vi "GetLowPrioritySensors.vi"() -> ()   [LabVIEW 2020]
doc: "All low priority sensor reads should be placed in this VI."
uses:
  GlobalMiscellaneous.vi
  GlobalDriverStationData.vi
  GlobalDrivebase.vi
  GRNF_CTREMotor.vi
  <vilib>/Rock Robotics/WPI/ThirdParty/Phoenix-LabVIEW/Motor Controller/Get/CTRE_Phoenix_MotorController_GetTemperature.vi
  GRNF_Compressor.vi
panel:
  out "Pressure Change (psi/min)":dbl
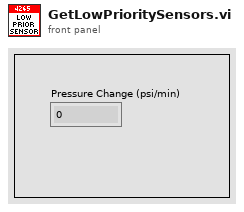
[diagram p1: front panel]
types:
  T1 = typedef "WPI_MotorControlDeviceRef.ctl" = cluster{"DeviceStatus":errorcluster, "Type":T2, "PWM":cluster{"PWM Channel":T3, "DeadBand":T4}, "CAN":cluster{"Device Number":u8, "SetOutput VI Ref":variant, "GetOutput VI Ref":variant, "Enable VI Ref":variant, "Disable VI Ref":variant, "Data":variant}, "Invert":bool, "DIO PWM":cluster{"PWM \"Enable\" Channel":T3, "DIOChannel":T5, "PWM Rate":dbl}}
  T2 = typedef "WPI_MotorControlType.ctl" = enum16{"PWM", "CAN", "DIO PWM"}
  T3 = typedef "FPGA_DIOPWMChannel.ctl" = enum8{"PWM 0", "PWM 1", "PWM 2", "PWM 3", "PWM 4", "PWM 5", "PWM 6", "PWM 7", "PWM 8", "PWM 9", "PWM MXP 0", "PWM MXP 1", "PWM MXP 2", "PWM MXP 3", "PWM MXP 4", "PWM MXP 5", "PWM MXP 6", "PWM MXP 7", "PWM MXP 8", "PWM MXP 9", "Invalid"}
  T4 = typedef "WPI_PWMDeadband.ctl" = cluster{"Name":string, "maxPositivePwm":i32, "minPositivePwm":i32, "centerPwm":i32, "maxNegativePwm":i32, "minNegativePwm":i32, "angularRange":u16}
  T5 = typedef "FPGA_DIOChannel.ctl" = enum8{"DIO 0", "DIO 1", "DIO 2", "DIO 3", "DIO 4", "DIO 5", "DIO 6", "DIO 7", "DIO 8", "DIO 9", "DIO MXP 0", "DIO MXP 1", "DIO MXP 2", "DIO MXP 3", "DIO MXP 4", "DIO MXP 5", "DIO MXP 6", "DIO MXP 7", "DIO MXP 8", "DIO MXP 9", "DIO MXP 10", "DIO MXP 11", "DIO MXP 12", "DIO MXP 13", "DIO MXP 14", "DIO MXP 15", "SPI Port CS1", "SPI Port CS2", "SPI Port CS3", "SPI Port MISO", "SPI Port MOSI", "Invalid"}
  T6 = typedef "WPI_CompressorDevRef.ctl" = cluster{"DevStatus":errorcluster, "Pneumatics Control Module":u8}
  T7 = cluster{"Pressure 0 (psi)":dbl, "Pressure 1 (psi)":dbl}
  T8 = cluster{"Battery Voltage Fault":bool, "Hardware Fault":bool, "CAN Warning Fault":bool, "Temperature Fault":bool}
  T9 = cluster{"HardwareFault":bool, "CompressorFault":bool, "SolenoidFault":bool, "Compressor Open":bool, "Brownout":bool}
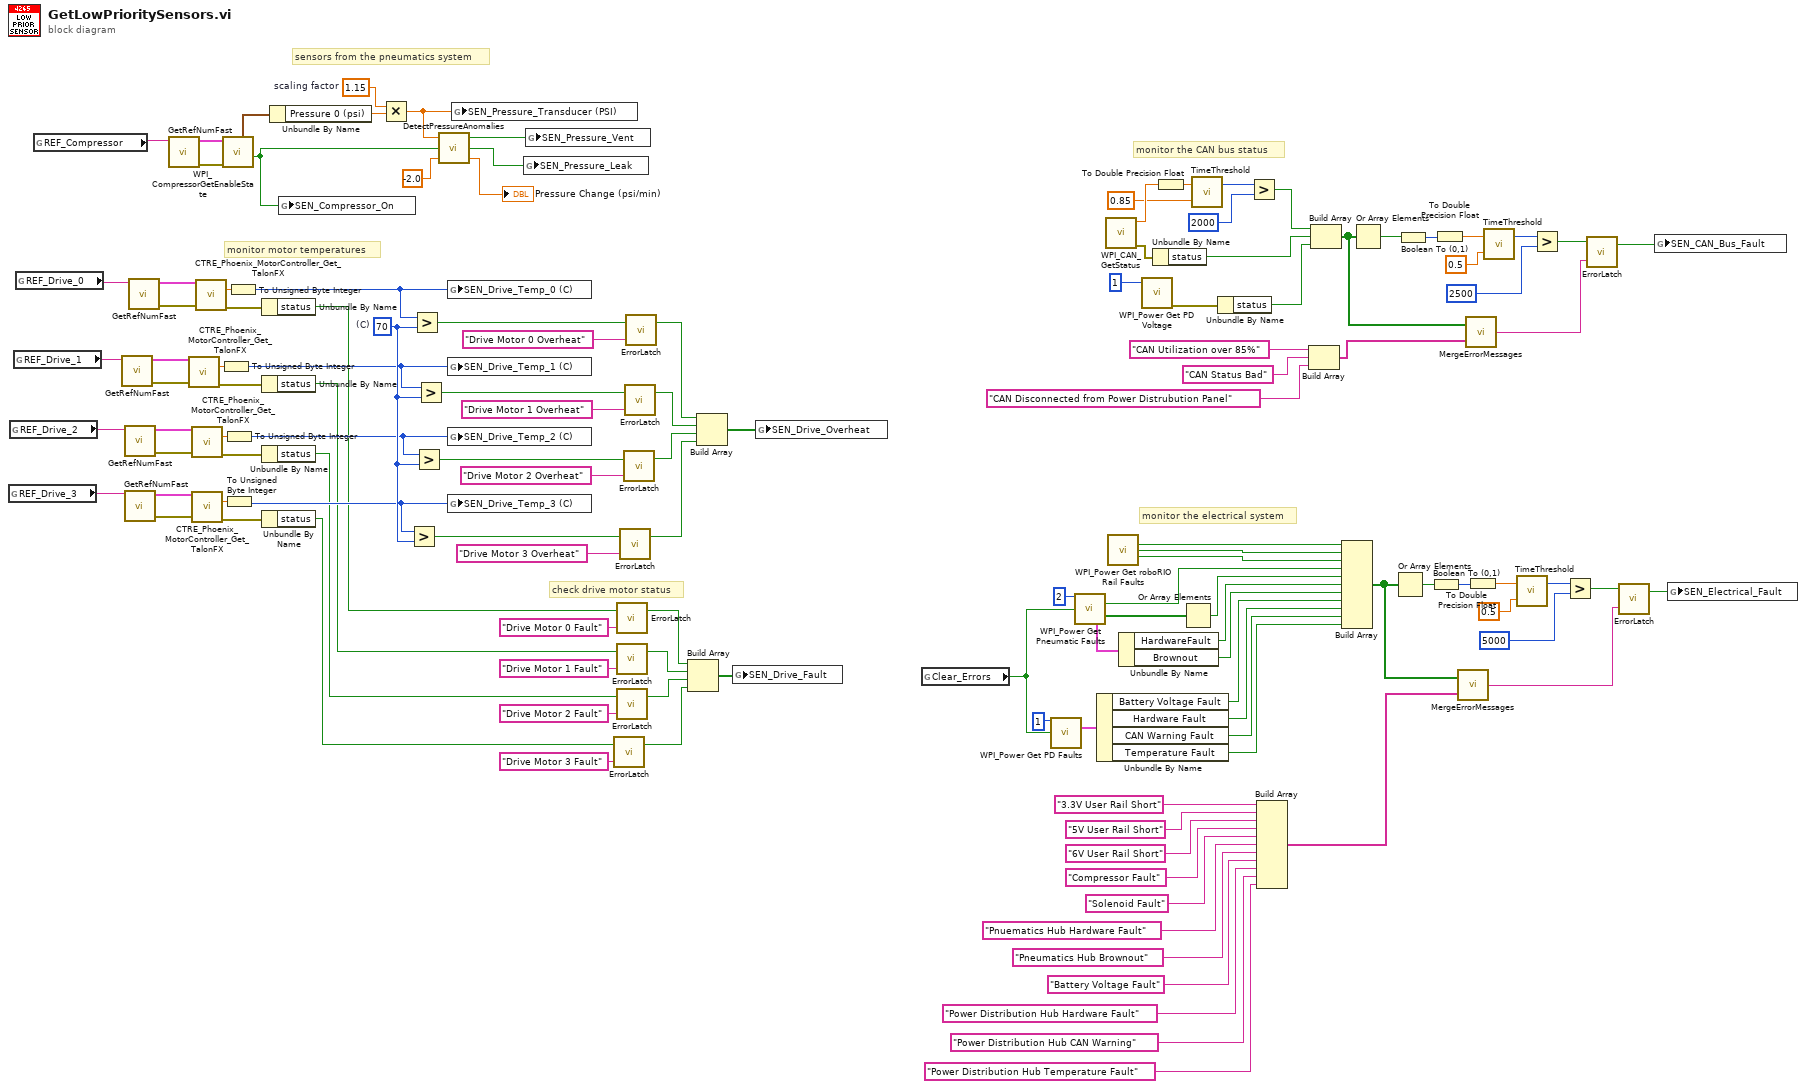
[diagram p0: block diagram]
diagram:
  w20 = 1.15  # scaling factor
  w127 = u8 70  # (C)
  # "check drive motor status"
  # "monitor the electrical system"
  # "monitor the CAN bus status"
  # "monitor motor temperatures"
  # "sensors from the pneumatics system"
  n1 = global read "GlobalDrivebase.vi" "REF_Drive_3"() -> (w71:string)
  n2 = global read "GlobalDrivebase.vi" "REF_Drive_2"() -> (w72:string)
  n3 = global read "GlobalDrivebase.vi" "REF_Drive_1"() -> (w73:string)
  n4 = global read "GlobalDrivebase.vi" "REF_Drive_0"() -> (w74:string)
  n5 = global read "GlobalMiscellaneous.vi" "REF_Compressor"() -> (w70:string)
  n6 = call-poly "GetRefNumFast.vi"("RefNum Name"=w73) -> ("Error"=w121:errorcluster, "Device Reference"=w122:T1)  [unwired: 5 in]
  n7 = call-poly "GetRefNumFast.vi"("RefNum Name"=w72) -> ("Error"=w118:errorcluster, "Device Reference"=w119:T1)  [unwired: 5 in]
  n8 = call-poly "GetRefNumFast.vi"("RefNum Name"=w71) -> ("Error"=w115:errorcluster, "Device Reference"=w116:T1)  [unwired: 5 in]
  n9 = call-poly "GetRefNumFast.vi"("RefNum Name"=w74) -> ("Error"=w124:errorcluster, "Device Reference"=w125:T1)  [unwired: 5 in]
  n10 = call-poly "GetRefNumFast.vi"("RefNum Name"=w70) -> ("Error"=w98:errorcluster, "Device Reference"=w99:T6)  [unwired: 5 in]
  n11 = call-poly <vilib>:"CTRE_Phoenix_MotorController_Get_TalonFX.vi"("PhoenixMotorControlDevRef"=w122, "error in"=w121) -> ("Temperature (C)"=w120:dbl, "error out"=w12:errorcluster)  [unwired: 11 in, 1 out]
  n12 = call-poly <vilib>:"CTRE_Phoenix_MotorController_Get_TalonFX.vi"("PhoenixMotorControlDevRef"=w119, "error in"=w118) -> ("Temperature (C)"=w117:dbl, "error out"=w11:errorcluster)  [unwired: 11 in, 1 out]
  n13 = call-poly <vilib>:"CTRE_Phoenix_MotorController_Get_TalonFX.vi"("PhoenixMotorControlDevRef"=w116, "error in"=w115) -> ("Temperature (C)"=w114:dbl, "error out"=w10:errorcluster)  [unwired: 11 in, 1 out]
  n14 = call-poly <vilib>:"CTRE_Phoenix_MotorController_Get_TalonFX.vi"("PhoenixMotorControlDevRef"=w125, "error in"=w124) -> ("Temperature (C)"=w123:dbl, "error out"=w13:errorcluster)  [unwired: 11 in, 1 out]
  n15 = To Unsigned Byte Integer(number=w120) -> (unsigned 8bit integer=w68:u8)
  n16 = call <vilib>:"WPI_CompressorGetEnableState.vi"("error in (no error)"=w98, "CompressorDevRef"=w99) -> ("Compressor Running"=w63:bool, "Pressure Sensors"=w80:T7)  [unwired: 3 in, 5 out]
  n17 = To Unsigned Byte Integer(number=w117) -> (unsigned 8bit integer=w67:u8)
  n18 = To Unsigned Byte Integer(number=w114) -> (unsigned 8bit integer=w66:u8)
  n19 = To Unsigned Byte Integer(number=w123) -> (unsigned 8bit integer=w69:u8)
  n20 = Unbundle By Name(w13) -> ("status"=w1:bool)
  n21 = Unbundle By Name(w12) -> ("status"=w7:bool)
  n22 = Unbundle By Name(w11) -> ("status"=w6:bool)
  n23 = Unbundle By Name(w10) -> ("status"=w5:bool)
  n24 = Unbundle By Name(w80) -> ("Pressure 0 (psi)"=w22:dbl)
  n25 = global write "GlobalMiscellaneous.vi" "SEN_Compressor_On"(w63) -> ()
  n26 = Multiply(x=w20, y=w22) -> (x*y=w21:dbl)
  n27 = Greater?(x=w66, y=w127) -> (0:w24:bool)
  n28 = Greater?(x=w69, y=w127) -> (0:w34:bool)
  n29 = Greater?(x=w67, y=w127) -> (0:w27:bool)
  n30 = Greater?(x=w68, y=w127) -> (0:w30:bool)
  n31 = call "DetectPressureAnomalies.vi"("Pressure Loss Threshold (psi/min)"=-2.0, "Compressor Running"=w63, "Pressure (psi)"=w21) -> ("Pressure Change (psi/min)"=→"Pressure Change (psi/min)":dbl, "Pressure Leak"=w64:bool, "Pressure Vent"=w65:bool)
  n32 = global write "GlobalDrivebase.vi" "SEN_Drive_Temp_0 (C)"(w69) -> ()
  n33 = global write "GlobalDrivebase.vi" "SEN_Drive_Temp_1 (C)"(w68) -> ()
  n34 = global write "GlobalDrivebase.vi" "SEN_Drive_Temp_2 (C)"(w67) -> ()
  n35 = global write "GlobalDrivebase.vi" "SEN_Drive_Temp_3 (C)"(w66) -> ()
  n36 = global write "GlobalMiscellaneous.vi" "SEN_Pressure_Transducer (PSI)"(w21) -> ()
  n37 = global write "GlobalMiscellaneous.vi" "SEN_Pressure_Leak"(w64) -> ()
  n38 = global write "GlobalMiscellaneous.vi" "SEN_Pressure_Vent"(w65) -> ()
  n39 = call "ErrorLatch.vi"("Error Message"="Drive Motor 3 Fault", "Trigger"=w5) -> ("Latched"=w8:bool)  [unwired: 1 in]
  n40 = call "ErrorLatch.vi"("Error Message"="Drive Motor 0 Fault", "Trigger"=w1) -> ("Latched"=w16:bool)  [unwired: 1 in]
  n41 = call "ErrorLatch.vi"("Error Message"="Drive Motor 1 Fault", "Trigger"=w7) -> ("Latched"=w15:bool)  [unwired: 1 in]
  n42 = call "ErrorLatch.vi"("Error Message"="Drive Motor 2 Fault", "Trigger"=w6) -> ("Latched"=w14:bool)  [unwired: 1 in]
  n43 = call "ErrorLatch.vi"("Error Message"="Drive Motor 3 Overheat", "Trigger"=w24) -> ("Latched"=w23:bool)  [unwired: 1 in]
  n44 = call "ErrorLatch.vi"("Error Message"="Drive Motor 2 Overheat", "Trigger"=w27) -> ("Latched"=w26:bool)  [unwired: 1 in]
  n45 = call "ErrorLatch.vi"("Error Message"="Drive Motor 1 Overheat", "Trigger"=w30) -> ("Latched"=w29:bool)  [unwired: 1 in]
  n46 = call "ErrorLatch.vi"("Error Message"="Drive Motor 0 Overheat", "Trigger"=w34) -> ("Latched"=w33:bool)  [unwired: 1 in]
  n47 = Build Array(w16, w15, w14, w8) -> (w4:bool[])
  n48 = Build Array(w33, w29, w26, w23) -> (w35:bool[])
  n49 = global write "GlobalDrivebase.vi" "SEN_Drive_Fault"(w4) -> ()
  n50 = global write "GlobalDrivebase.vi" "SEN_Drive_Overheat"(w35) -> ()
  n51 = global read "GlobalDriverStationData.vi" "Clear_Errors"() -> (w81:bool)
  n52 = call <vilib>:"WPI_Power Get PD Faults.vi"("Power Distribution (def)"=u8 1, "Clear Sticky Faults"=w81) -> ("Faults"=w91:T8)  [unwired: 10 in, 3 out]
  n53 = call <vilib>:"WPI_Power Get Pneumatic Faults.vi"("Pneumatics device (def)"=u8 2, "Clear Sticky Faults"=w81) -> ("Compressor Fault"=w96:bool, "All Solenoid Faults"=w95:bool[], "Faults"=w87:T9)  [unwired: 8 in, 3 out]
  n54 = Unbundle By Name(w91) -> ("Battery Voltage Fault"=w36:bool, "Hardware Fault"=w84:bool, "CAN Warning Fault"=w83:bool, "Temperature Fault"=w82:bool)
  n55 = call <vilib>:"WPI_CAN_GetStatus.vi"() -> ("error out"=w113:errorcluster, "Percent Bus Utilization"=w110:sgl)  [unwired: 6 in, 4 out]
  n56 = call <vilib>:"WPI_Power Get roboRIO Rail Faults.vi"() -> ("3.3V User Rail Short"=w94:bool, "5 V User Rail Short"=w93:bool, "6 V User Rail Short"=w92:bool)  [unwired: 10 in, 3 out]
  n57 = Unbundle By Name(w87) -> ("HardwareFault"=w86:bool, "Brownout"=w85:bool)
  n58 = call <vilib>:"WPI_Power Get PD Voltage.vi"("Power Distribution Panel (def)"=u8 1 ("Power Distribution Panel (0)")) -> ("error out"=w89:errorcluster)  [unwired: 13 in, 1 out]
  n59 = Unbundle By Name(w113) -> ("status"=w112:bool)
  n60 = To Double Precision Float(number=w110) -> (double precision float=w108:dbl)
  n61 = Or Array Elements(Boolean array=w95) -> (logical OR=w126:bool)
  n62 = call "TimeThreshold.vi"("Threshold"=0.85, "Current Value"=w108) -> ("Time Above Threshold (ms)"=w107:u32)  [unwired: 1 out]
  n63 = Unbundle By Name(w89) -> ("status"=w111:bool)
  n64 = Greater?(x=w107, y=u32 2000) -> (0:w2:bool)
  n65 = Build Array("3.3V User Rail Short", "5V User Rail Short" ("element"), "6V User Rail Short" ("element"), "Compressor Fault" ("element"), "Solenoid Fault" ("element"), "Pnuematics Hub Hardware Fault" ("element"), "Pneumatics Hub Brownout" ("element"), "Battery Voltage Fault" ("element"), "Power Distribution Hub Hardware Fault" ("element"), "Power Distribution Hub CAN Warning" ("element"), "Power Distribution Hub Temperature Fault" ("element")) -> (w41:string[])
  n66 = Build Array("CAN Utilization over 85%", "CAN Status Bad" ("element"), "CAN Disconnected from Power Distrubution Panel" ("element")) -> (w37:string[])
  n67 = Build Array(w2, w112, w111) -> (w38:bool[])
  n68 = Build Array(w94, w93, w92, w96, w126, w86, w85, w36, w84, w83, w82) -> (w40:bool[])
  n69 = Or Array Elements(Boolean array=w38) -> (logical OR=w42:bool)
  n70 = Or Array Elements(Boolean array=w40) -> (logical OR=w60:bool)
  n71 = Boolean To (0,1)(Boolean=w42) -> (0, 1=w79:i16)
  n72 = Boolean To (0,1)(Boolean=w60) -> (0, 1=w106:i16)
  n73 = To Double Precision Float(number=w79) -> (double precision float=w78:dbl)
  n74 = call "MergeErrorMessages.vi"("Error Descriptions"=w41, "Active Errors"=w40) -> ("Merged Error Message"=w48:string)
  n75 = call "MergeErrorMessages.vi"("Error Descriptions"=w37, "Active Errors"=w38) -> ("Merged Error Message"=w39:string)
  n76 = To Double Precision Float(number=w106) -> (double precision float=w105:dbl)
  n77 = call "TimeThreshold.vi"("Threshold"=0.5, "Current Value"=w78) -> ("Time Above Threshold (ms)"=w76:u32)  [unwired: 1 out]
  n78 = call "TimeThreshold.vi"("Threshold"=0.5, "Current Value"=w105) -> ("Time Above Threshold (ms)"=w103:u32)  [unwired: 1 out]
  n79 = Greater?(x=w76, y=u32 2500) -> (0:w44:bool)
  n80 = Greater?(x=w103, y=u32 5000) -> (0:w62:bool)
  n81 = call "ErrorLatch.vi"("Error Message"=w39, "Trigger"=w44) -> ("Latched"=w43:bool)  [unwired: 1 in]
  n82 = call "ErrorLatch.vi"("Error Message"=w48, "Trigger"=w62) -> ("Latched"=w61:bool)  [unwired: 1 in]
  n83 = global write "GlobalMiscellaneous.vi" "SEN_CAN_Bus_Fault"(w43) -> ()
  n84 = global write "GlobalMiscellaneous.vi" "SEN_Electrical_Fault"(w61) -> ()
